vi "mainSC.vi"(11 "extraplots":T1) -> ()   [LabVIEW 2014]
uses:
  controlSC.ctl
  dataSC.ctl
panel:
  out "extras":cluster{"x":dbl[], "y":dbl[]}[](graph)
  in  "scale":dbl
  out "unity circle":cluster{"x":dbl[], "y":dbl[]}[](graph)
  in  "plot":bool
  out "R":cluster{"x":dbl[], "y":dbl[]}[](graph)
  out "X":cluster{"x":dbl[], "y":dbl[]}[](graph)
  in  "stop":bool
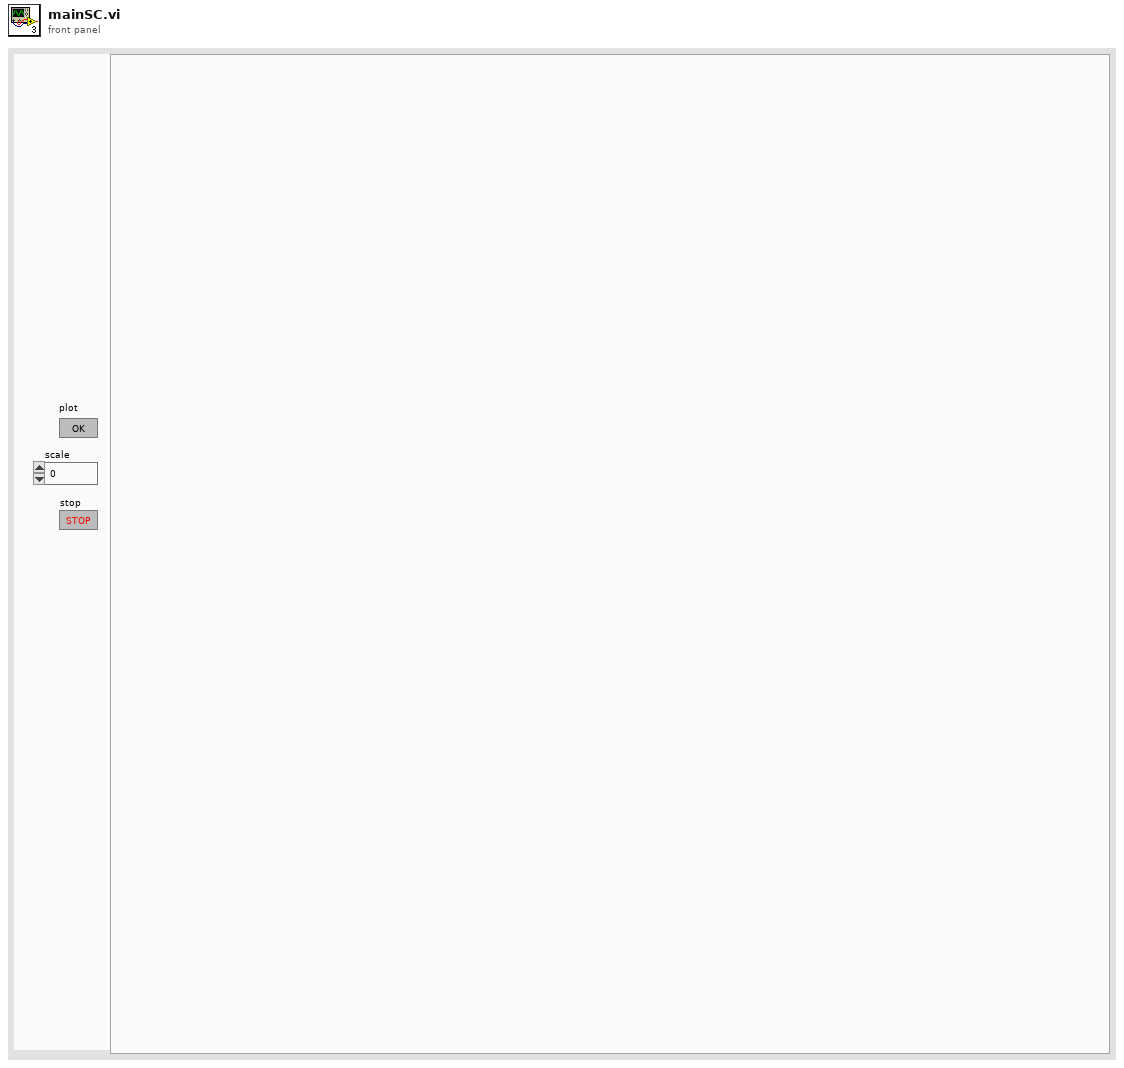
[diagram p1: front panel]
types:
  T1 = cluster{"1":cdb[], "2":cdb[], "3":cdb[], "4":cdb[], "5":cdb[]}
  T2 = typedef "dataSC.ctl" = cluster{"allplots":cluster{"x":dbl[], "y":dbl[]}[], "extra":cluster{"indexes":i32[], "allextras":dbl[][]}, "scale":dbl, "extraplots":cluster{"Array":cdb[], "Array 2":cdb[], "Array 3":cdb[], "Array 4":cdb[], "Array 5":cdb[]}, "loops":i32, "extras":cluster{"Array":dbl[], "Array 2":dbl[]}[], "unitycircle":cluster{"Array":dbl[], "Array 2":dbl[]}[], "R":cluster{"Array":dbl[], "Array 2":dbl[]}[], "X":cluster{"Array":dbl[], "Array 2":dbl[]}[]}
  T3 = typedef "controlSC.ctl" = enum16{"idle", "extract data", "unity circle", "smith chart", "plot", "configure extras", "configure unity circle", "configure R", "configure X"}
  T4 = cluster{"Array":cdb[], "Array 2":cdb[], "Array 3":cdb[], "Array 4":cdb[], "Array 5":cdb[]}
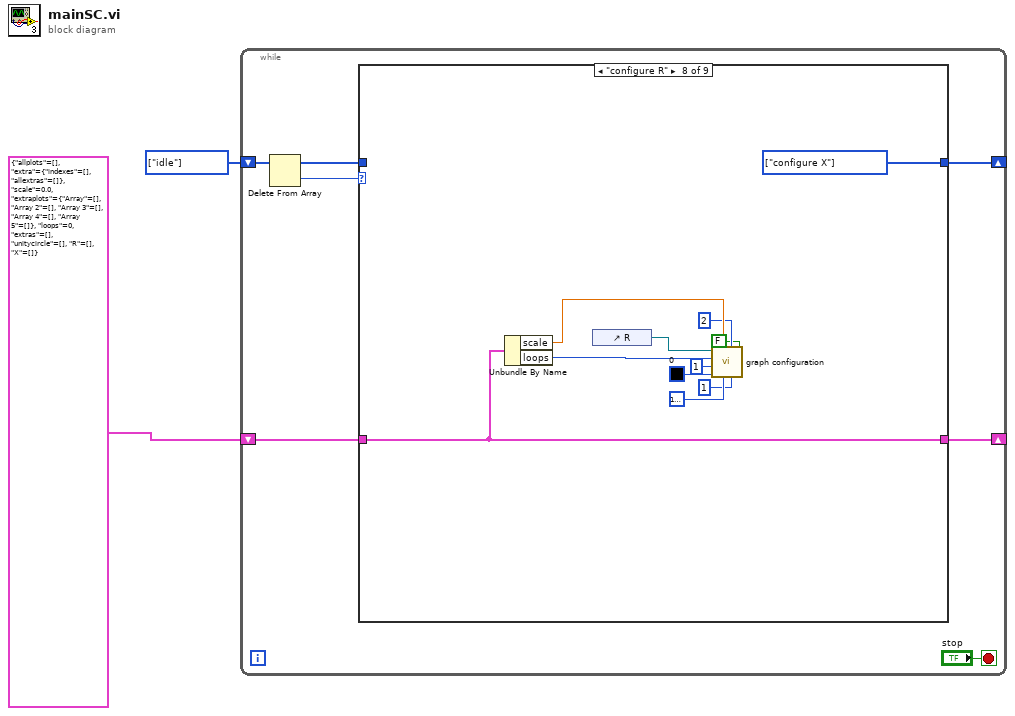
[diagram p0: block diagram]
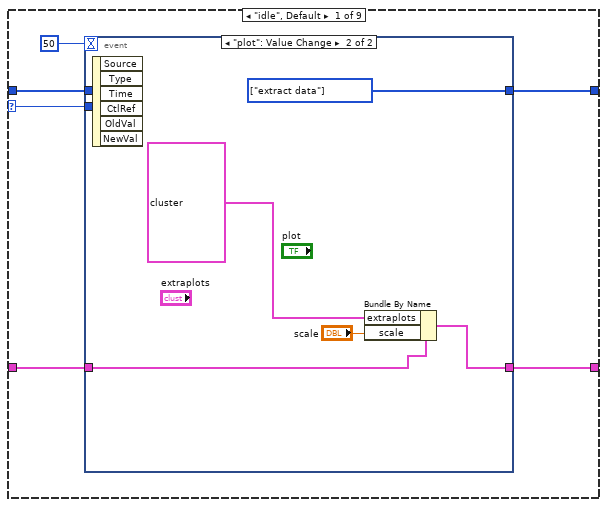
[diagram p2: hidden frame]
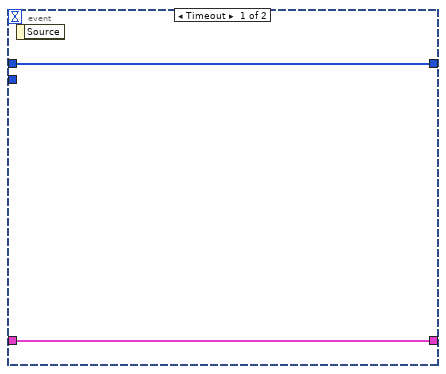
[diagram p3: hidden frame]
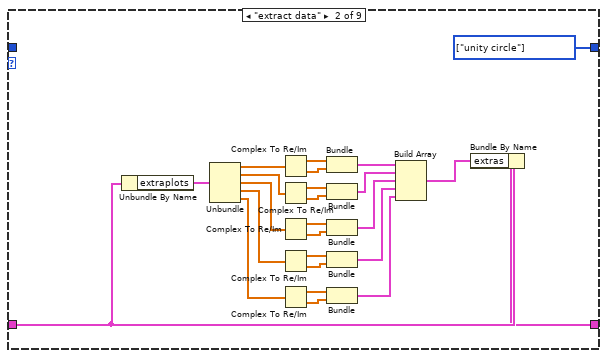
[diagram p4: hidden frame]
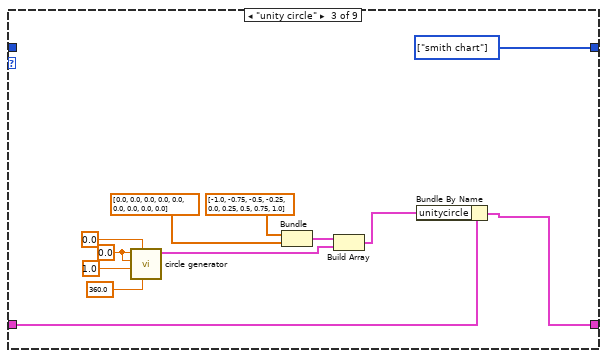
[diagram p5: hidden frame]
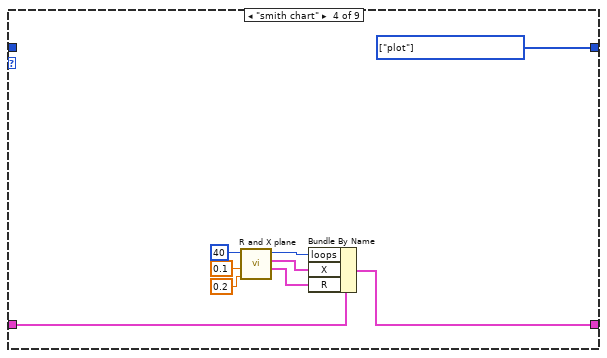
[diagram p6: hidden frame]
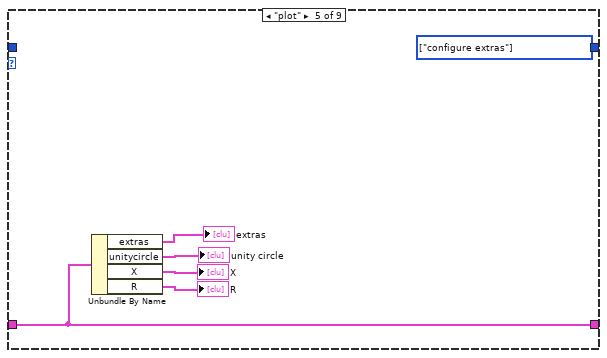
[diagram p7: hidden frame]
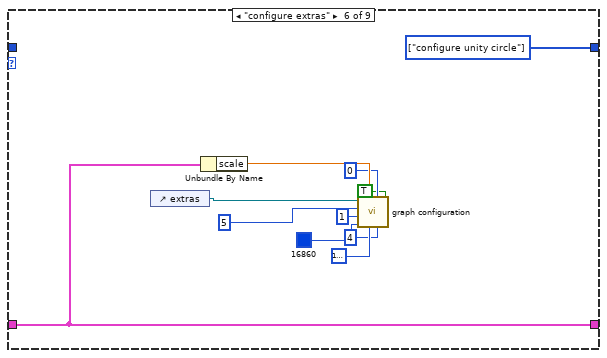
[diagram p8: hidden frame]
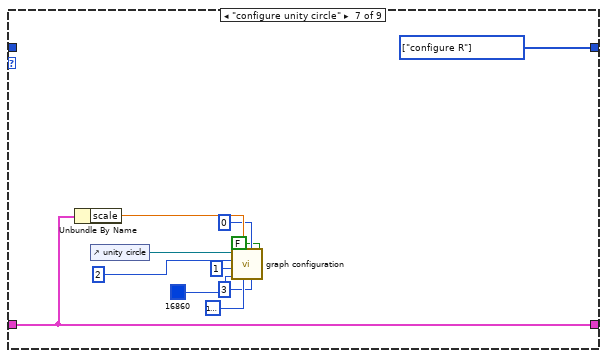
[diagram p9: hidden frame]
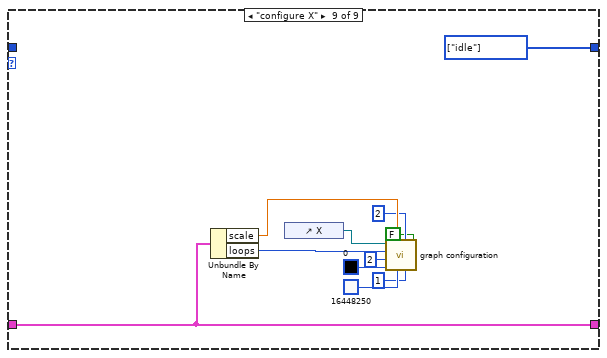
[diagram p10: hidden frame]
diagram:
  w2 = T3[] [enum."idle"] items=["idle", "extract data", "unity circle", "smith chart", "plot", "configure extras", "configure unity circle", "configure R", "configure X"]
  n1 = while {
    shift-right: [w6] -> _
    shift-left: w2 -> [w9]
    shift-right: [w5] -> _
    shift-left: T2 {"allplots"=[], "extra"={"indexes"=[], "allextras"=[]}, "scale"=0.0, "extraplots"={"Array"=[], "Array 2"=[], "Array 3"=[], "Array 4"=[], "Array 5"=[]}, "loops"=0, "extras"=[], "unitycircle"=[], "R"=[], "X"=[]} ("data") -> [w3]
    stop <- "stop" stop-if-true
    n2 = Delete From Array(array=w9) -> (deleted portion=w8:T3, array with subset deleted=w7:T3[])  [unwired: 2 in]
    n3 = case shown="\"configure R\"" w8 {
      selector: w8 -> [w13 _ _ _ _ _ _ _ _]
      tunnel: w7 -> [w14 _ _ _ _ _ _ _ _]
      tunnel: [w12 w46 w50 w68 w72 w76 w91 w103 w115] -> w6
      tunnel: w3 -> [w10 w24 w49 w61 w69 w75 w86 w97 w108]
      tunnel: [w11 w23 w48 w60 w69 w75 w86 w97 w108] -> w5
      frame "idle", Default {
        n4 = event shown="[1] \"plot\": Value Change" {
          selector: _ -> [_ _]
          dyn-events: _ -> [_ _]
          timeout: 50 -> [_ _]
          tunnel: w14 -> [w17 _]
          tunnel: w13 -> [_ _]
          tunnel: [w17 w22] -> w12
          tunnel: [w16 w19] -> w11
          tunnel: w10 -> [w16 w20]
          event Timeout {
            n5 = event-data() -> ()  [unwired: 1 in, 1 out]
          }
          event "plot": Value Change {
            w22 = T3[] [enum."extract data"] items=["idle", "extract data", "unity circle", "smith chart", "plot", "configure extras", "configure unity circle", "configure R", "configure X"]
            n6 = event-data() -> ()  [unwired: 1 in, 6 out]
            n7 = Bundle By Name(cluster=w20, "extraplots"=cluster{cdb[], cdb[], cdb[], cdb[], cdb[]} {array[360 elements], array[360 elements], array[360 elements], array[360 elements], array[360 elements]} ("output cluster"), "scale"="scale") -> (w19:T2)
          }
        }
      }
      frame "extract data" {
        w46 = T3[] [enum."unity circle"] items=["idle", "extract data", "unity circle", "smith chart", "plot", "configure extras", "configure unity circle", "configure R", "configure X"]
        n8 = Unbundle By Name(w24) -> ("extraplots"=w47:T4)
        n9 = Unbundle(w47) -> ("Array"=w45:cdb[], "Array 2"=w44:cdb[], "Array 3"=w43:cdb[], "Array 4"=w42:cdb[], "Array 5"=w41:cdb[])
        n10 = Complex To Re/Im(x + iy=w45) -> (x=w40:dbl[], y=w39:dbl[])
        n11 = Complex To Re/Im(x + iy=w44) -> (x=w38:dbl[], y=w37:dbl[])
        n12 = Complex To Re/Im(x + iy=w43) -> (x=w36:dbl[], y=w35:dbl[])
        n13 = Complex To Re/Im(x + iy=w42) -> (x=w34:dbl[], y=w33:dbl[])
        n14 = Complex To Re/Im(x + iy=w41) -> (x=w32:dbl[], y=w31:dbl[])
        n15 = Bundle(w40, w39) -> (w30:cluster{dbl[], dbl[]})  [unwired: 1 in]
        n16 = Bundle(w38, w37) -> (w29:cluster{dbl[], dbl[]})  [unwired: 1 in]
        n17 = Bundle(w36, w35) -> (w28:cluster{dbl[], dbl[]})  [unwired: 1 in]
        n18 = Bundle(w34, w33) -> (w27:cluster{dbl[], dbl[]})  [unwired: 1 in]
        n19 = Bundle(w32, w31) -> (w26:cluster{dbl[], dbl[]})  [unwired: 1 in]
        n20 = Build Array(w30, w29, w28, w27, w26) -> (w25:cluster{dbl[], dbl[]}[])
        n21 = Bundle By Name(cluster=w24, "extras"=w25) -> (w23:T2)
      }
      frame "unity circle" {
        w50 = T3[] [enum."smith chart"] items=["idle", "extract data", "unity circle", "smith chart", "plot", "configure extras", "configure unity circle", "configure R", "configure X"]
        w55 = 0.0 ("r 2")
        n22 = call "circle generator.vi"("end"=360.0, "start"=0.0, "r"=1.0 ("r 2"), "yc"=w55, "xc"=w55) -> ("graph"=w59:cluster{dbl[], dbl[]})  [unwired: 4 in, 2 out]
        n23 = Bundle(dbl[] [-1.0, -0.75, -0.5, -0.25, 0.0, 0.25, 0.5, 0.75, 1.0], dbl[] [0.0, 0.0, 0.0, 0.0, 0.0, 0.0, 0.0, 0.0, 0.0]) -> (w54:cluster{dbl[], dbl[]})  [unwired: 1 in]
        n24 = Build Array(w54, w59) -> (w51:cluster{dbl[], dbl[]}[])
        n25 = Bundle By Name(cluster=w49, "unitycircle"=w51) -> (w48:T2)
      }
      frame "smith chart" {
        w68 = T3[] [enum."plot"] items=["idle", "extract data", "unity circle", "smith chart", "plot", "configure extras", "configure unity circle", "configure R", "configure X"]
        n26 = call "R and X plane.vi"("inc"=0.2, "R0,X0"=0.1, "loops"=40) -> ("R"=w62:cluster{dbl[], dbl[]}[], "X"=w63:cluster{"x":dbl[], dbl[]}[], "loops"=w64:i32)  [unwired: 6 in]
        n27 = Bundle By Name(cluster=w61, "loops"=w64, "X"=w63, "R"=w62) -> (w60:T2)
      }
      frame "plot" {
        w72 = T3[] [enum."configure extras"] items=["idle", "extract data", "unity circle", "smith chart", "plot", "configure extras", "configure unity circle", "configure R", "configure X"]
        n28 = Unbundle By Name(w69) -> ("extras"=→"extras":cluster{"Array":dbl[], "Array 2":dbl[]}[], "unitycircle"=→"unity circle":cluster{"Array":dbl[], "Array 2":dbl[]}[], "X"=→"X":cluster{"Array":dbl[], "Array 2":dbl[]}[], "R"=→"R":cluster{"Array":dbl[], "Array 2":dbl[]}[])
      }
      frame "configure extras" {
        w76 = T3[] [enum."configure unity circle"] items=["idle", "extract data", "unity circle", "smith chart", "plot", "configure extras", "configure unity circle", "configure R", "configure X"]
        n29 = control-ref of="extras"() -> (w78:refnum<vi>)
        n30 = Unbundle By Name(w75) -> ("scale"=w81:dbl)
        n31 = call "graph configuration.vi"("extras?"=TRUE, "width"=u8 4, "style"=u8 0, "BG"=u32 16777216, "scale"=w81, "line color"=u32 16860, "multiplicator"=1, "loops"=5, "graph"=w78) -> ()  [unwired: 3 in]
      }
      frame "configure unity circle" {
        w91 = T3[] [enum."configure R"] items=["idle", "extract data", "unity circle", "smith chart", "plot", "configure extras", "configure unity circle", "configure R", "configure X"]
        n32 = Unbundle By Name(w86) -> ("scale"=w90:dbl)
        n33 = control-ref of="unity circle"() -> (w93:refnum<vi>)
        n34 = call "graph configuration.vi"("extras?"=FALSE, "width"=u8 3, "style"=u8 0, "BG"=u32 16777216, "scale"=w90, "line color"=u32 16860, "multiplicator"=1, "loops"=2, "graph"=w93) -> ()  [unwired: 3 in]
      }
      frame "configure R" {
        w103 = T3[] [enum."configure X"] items=["idle", "extract data", "unity circle", "smith chart", "plot", "configure extras", "configure unity circle", "configure R", "configure X"]
        n35 = Unbundle By Name(w97) -> ("scale"=w101:dbl, "loops"=w106:i32)
        n36 = control-ref of="R"() -> (w107:refnum<vi>)
        n37 = call "graph configuration.vi"("extras?"=FALSE, "width"=u8 1, "style"=u8 2, "BG"=u32 16777216, "scale"=w101, "line color"=u32 0, "multiplicator"=1, "loops"=w106, "graph"=w107) -> ()  [unwired: 3 in]
      }
      frame "configure X" {
        w115 = T3[] [enum."idle"] items=["idle", "extract data", "unity circle", "smith chart", "plot", "configure extras", "configure unity circle", "configure R", "configure X"]
        n38 = Unbundle By Name(w108) -> ("scale"=w112:dbl, "loops"=w118:i32)
        n39 = control-ref of="X"() -> (w114:refnum<vi>)
        n40 = call "graph configuration.vi"("extras?"=FALSE, "width"=u8 1, "style"=u8 2, "BG"=u32 16448250, "scale"=w112, "line color"=u32 0, "multiplicator"=2, "loops"=w118, "graph"=w114) -> ()  [unwired: 3 in]
      }
    }
  }
